vi "SetChartParams.vi"(8 "error in (no error)":errorcluster, 10 "ChartParams":T1={"Chart ScaleMultipliers"={"WF Xscale Multiplier"=0.0, "WF Yscale Multiplier"=[]}, "Coord Transform Multipliers"={"Z-Multiplier"=1.0, "Th-Multiplier"=0.0}}, 11 "DisplayWaveforms":refnum<class "DisplayWaveforms.lvclass">) -> (0 "error out":errorcluster, 3 "DisplayWaveforms out":refnum<class "DisplayWaveforms.lvclass">)   [LabVIEW 2020, in "DisplayWaveform.lvlib" / "DisplayWaveforms.lvclass"]
doc: "Set Chart Attributes"
uses:
  DisplayWaveforms.lvclass
  Controller/TypeDefs/ChartParamsCluster.ctl
panel:
  # "For instructions on how to use the JKI State Machine Objects, examples and video tutorials, visit:\nhttp://jki.net/state-machine-objects/\n\nJKI State Machine Objects™\nhttp://jki.net/state-machine-objects/\nCopyright (C) 2005-2015, JKI <info@jki.net>\nALL RIGHTS RESERVED"
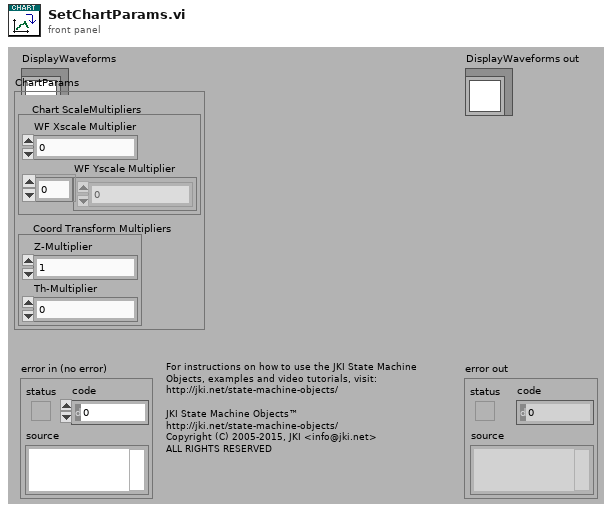
[diagram p1: front panel]
types:
  T1 = typedef "ChartParamsCluster.ctl" = cluster{"Chart ScaleMultipliers":cluster{"WF Xscale Multiplier":dbl, "WF Yscale Multiplier":dbl[]}, "Coord Transform Multipliers":cluster{"Z-Multiplier":dbl, "Th-Multiplier":dbl}}
  T2 = typedef "DisplayWaveform.lvlib/DisplayWaveforms.lvclass/ProtectedEvents--Cluster.ctl" = cluster{"Clear Chart":refnum<user-event>, "Pause Chart":refnum<user-event>, "Update Chart":refnum<user-event>, "Export Chart":refnum<user-event>, "Set ChartParams":refnum<user-event>}
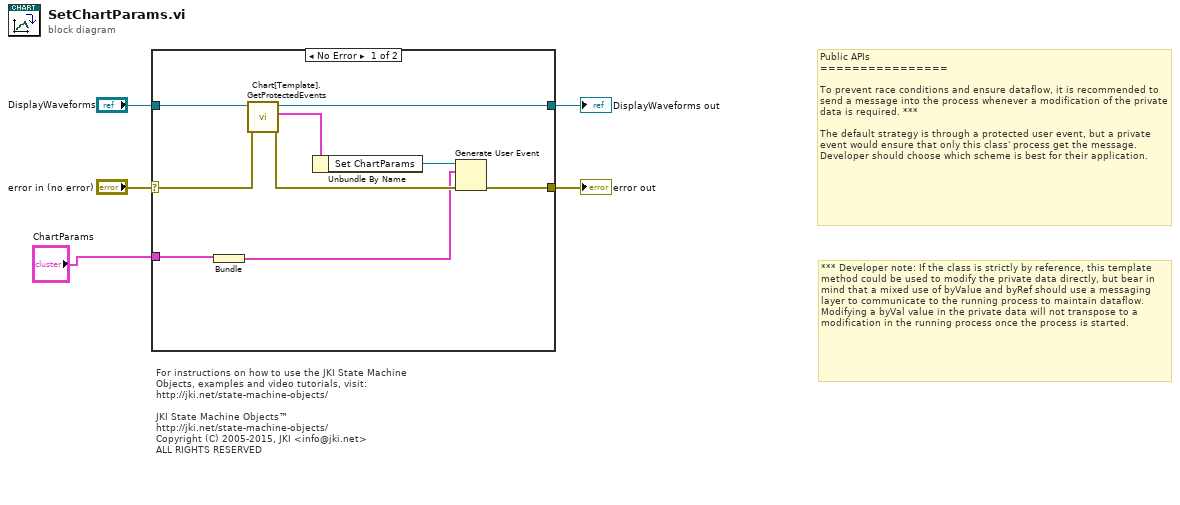
[diagram p0: block diagram]
diagram:
  # "*** Developer note: If the class is strictly by reference, this template method could be used to modify the private data directly, but bear in mind that a mixed use of byValue and byRef should use a messaging layer to communicate to the running process to maintain dataflow. Modifying a byVal value in the private data will not transpose to a modification in the running process once the process is started."
  # "Public APIs\n================\n\nTo prevent race conditions and ensure dataflow, it is recommended to send a message into the process whenever a modification of the private data is required. ***\n\nThe default strategy is through a protected user event, but a private event would ensure that only this class' process get the message. Developer should choose which scheme is best for their application."
  # "For instructions on how to use the JKI State Machine Objects, examples and video tutorials, visit:\nhttp://jki.net/state-machine-objects/\n\nJKI State Machine Objects™\nhttp://jki.net/state-machine-objects/\nCopyright (C) 2005-2015, JKI <info@jki.net>\nALL RIGHTS RESERVED"
  n1 = case shown="No Error" "error in (no error)" {
    selector: "error in (no error)" -> [w14 w15]
    tunnel: "DisplayWaveforms" -> [w11 w16]
    tunnel: [w13 w15] -> w4
    tunnel: [w12 w16] -> w3
    tunnel: "ChartParams" -> [w7 _]
    frame No Error {
      n2 = Bundle("ChartParams"=w7) -> (w6:cluster{"ChartParams":T1})  [unwired: 1 in]
      n3 = call "Chart[Template].GetProtectedEvents.vi"("error in (no error)"=w14, "DisplayWaveforms"=w11) -> ("error out"=w8:errorcluster, "Protected Events"=w9:T2, "DisplayWaveforms out"=w12:refnum<class "DisplayWaveforms.lvclass">)  [unwired: 7 in]
      n4 = Unbundle By Name(w9) -> ("Set ChartParams"=w10:refnum<user-event>)
      n5 = Generate User Event(user event=w10, event data cluster=w6, error in=w8) -> (error out=w13:errorcluster)  [unwired: 1 in, 1 out]
    }
    frame Error {
    }
  }
  "error out" <- w4
  "DisplayWaveforms out" <- w3
